vi "Manual.vi"(8 "error in (no error)":errorcluster, 10 "shutdown":refnum<user-event>, 11 "Modules":T1) -> (0 "Error 2":errorcluster)   [LabVIEW 2025]
uses:
  <vilib>/Handler Framework/CmdQueue/Enqueue Single.vi
  <vilib>/Handler Framework/Handler Framework.lvlib
panel:
  out "Module Names":string[](array[string])
  out "Error":errorcluster
  # "Diagnostics"
  # "Modules"
  # "USB I/O"
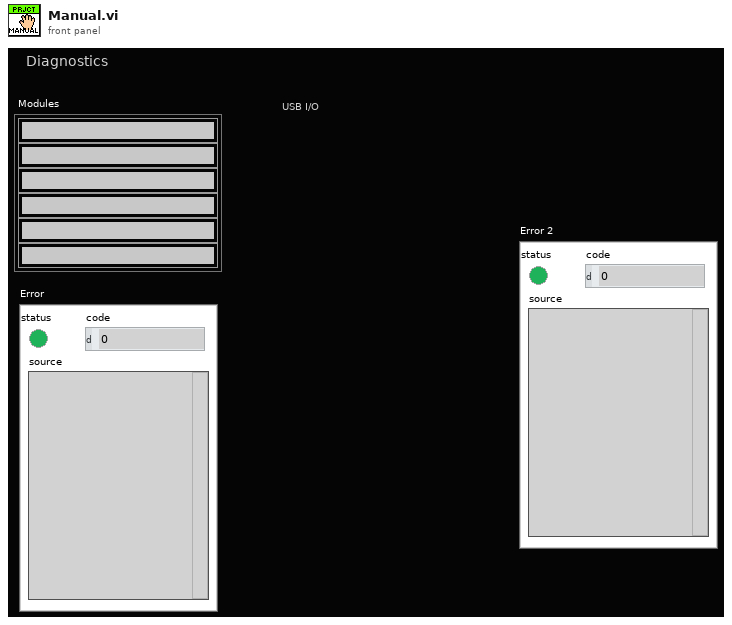
[diagram p1: front panel]
types:
  T1 = cluster{"Module IDs":i32[], "Module Names":string[]}
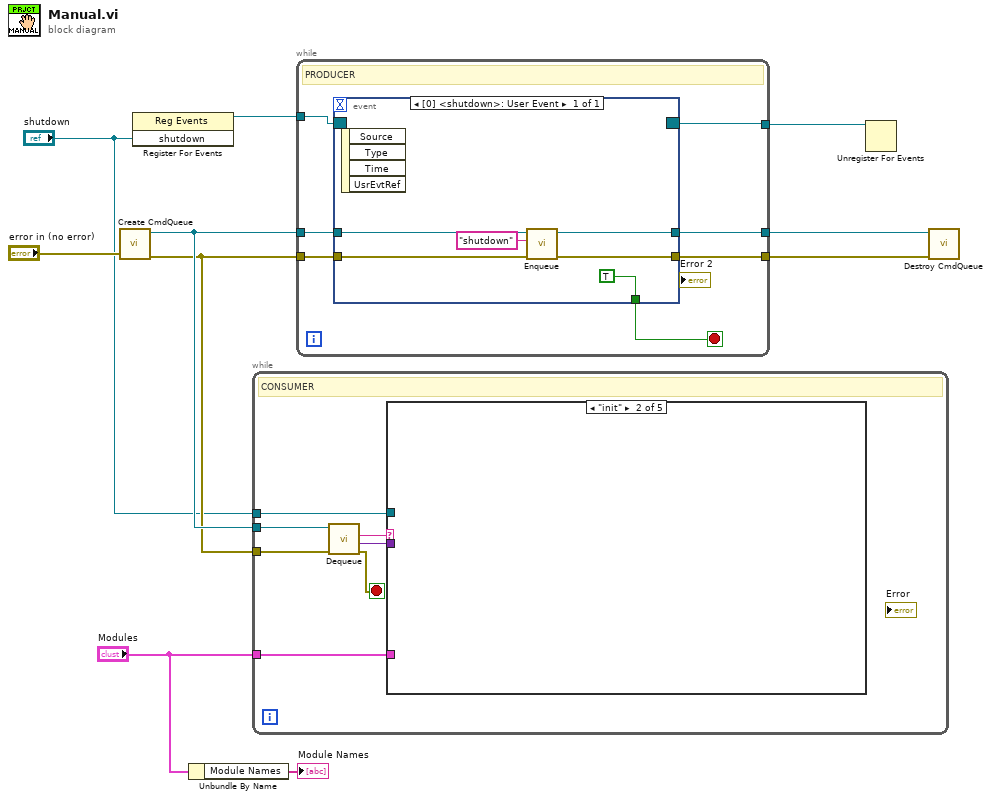
[diagram p0: block diagram]
diagram:
  n1 = call <vilib>:"Create CmdQueue.vi"("error in (no error)"="error in (no error)") -> ("error out"=w7:errorcluster, "CmdQueue out"=w8:refnum<queue>)  [unwired: 9 in]
  n2 = register-events("shutdown") -> (reference out=w6:refnum<event-registration>)  [unwired: 2 in, 1 out]
  n3 = Unbundle By Name("Modules") -> ("Module Names"=→"Module Names":string[])
  n4 = while {
    tunnel: w8 -> [w17]
    tunnel: w7 -> [w13]
    tunnel: "shutdown" -> [w12]
    tunnel: "Modules" -> [w11]
    stop <- w14 stop-if-true
    # "CONSUMER"
    n5 = call <vilib>:"Dequeue.vi"("error in (no error)"=w13, "CmdQueue in"=w17) -> ("error out"=w14:errorcluster, "value"=w15:variant, "cmd"=w16:string)  [unwired: 5 in, 2 out]
    n6 = case shown="\"init\"" w16 {
      tunnel: w15 -> [_ _ _ _ _]
      tunnel: w12 -> [_ _ _ _ _]
      tunnel: w11 -> [_ _ _ _ _]
      frame "False", Default {
      }
      frame "init" {
      }
      frame "shutdown" {
      }
      frame "append" {
      }
      frame "save & clear" {
      }
    }
  }
  n7 = while {
    tunnel: w8 -> [w24]
    tunnel: [w23] -> w10
    tunnel: w7 -> [w22]
    tunnel: [w21] -> w9
    tunnel: w6 -> [w19]
    tunnel: [w18] -> w5
    stop <- w20 stop-if-true
    # "PRODUCER"
    n8 = event shown="[0] <shutdown>: User Event" {
      selector: w19 -> [_]
      dyn-events: [_] -> w18
      timeout: _ -> [_]
      tunnel: w24 -> [w30]
      tunnel: [w29] -> w23
      tunnel: w22 -> [w28]
      tunnel: [w27] -> w21
      tunnel: [TRUE ("Discard?")] -> w20
      event User Event {
        n9 = event-data() -> ()  [unwired: 1 in, 4 out]
        n10 = call-poly <vilib>:"Enqueue.vi"("error in (no error)"=w28, "Command"="shutdown", "CmdQueue in"=w30) -> ("error out"=w27:errorcluster, "CmdQueue out"=w29:refnum<queue>)  [unwired: 7 in]
      }
    }
  }
  n11 = Unregister For Events(event registration refnum=w5) -> ()  [unwired: 1 in, 1 out]
  n12 = call <vilib>:"Destroy CmdQueue.vi"("error in (no error)"=w9, "CmdQueue in"=w10) -> ()  [unwired: 9 in, 1 out]
